vi "MARS_Global_var.vi"() -> ()   [LabVIEW 2015]
panel:
  in  "Fit Selection":bool
  in  "Int. Selector":bool caption="Integral Selector"
  in  "Select":bool
  in  "lower limit":i32
  in  "upper limit":i32
  in  "Listbox":i32[](array[numeric])
  out "Meas. Duration":dbl format="%^#.3g"
  out "2nd Integr.":dbl format="%^#.2g"
  out "1st Integr.":dbl format="%^#.2g"
  out "Trigger Level":dbl format="%#.3p"
  in  "Fit index":i32=1
  out "FoM":dbl
  out "Histogram":i32[][](graph)
  in  "Spectrum sel. 2":bool
  out "Discr. Spectrum":i32[][](array[numeric])
  out "Neutron Counts %":dbl format="%#.2f"
  out "Gamma Counts %":dbl format="%#.2f"
  out "Isotope Spectrum":i32[][](array[numeric])
  in  "Spectr. Sel.":bool
  out "Int Graph":i32[][](graph)
  out "Scatter":T1(graph) caption="Scatter Plot"
  out "Spectrum":i32[][](graph)
  out "Gamma Counts":i32
  out "Neutron Counts":i32
  out "Total Counts":i32
  in  "Fit Slope":dbl
  in  "Fit Offset":dbl
  out "Total Int. Auto":i32[][][](array[numeric])
  out "Tail Int. Auto":i32[][][](array[numeric])
  out "Total Integral":i32[](array[numeric])
  out "Tail Integral":i32[](array[numeric])
  out "Prog Ind":bool caption="CyUSB\nProg."
  out "Config Ind":bool caption="MB \nConfig."
  in  "Integ_per":cluster{dbl, dbl}(slide) caption="Duration of Integration (us)" scale=0.0..10.0
  in  "Error":errorcluster
  in  "Trig_thr":dbl(slide) caption="Trigger Threshold (V)" min=0.0 max=3.3 step=0.001 scale=0.0..3.3
  in  "CyUSB VISA":refnum<visa-resource-name>
  # "VISA Resource"
  # "Indicators"
  # "Configuration Data"
  # "Free Run Results Data"
  # "Auto Test Results Data"
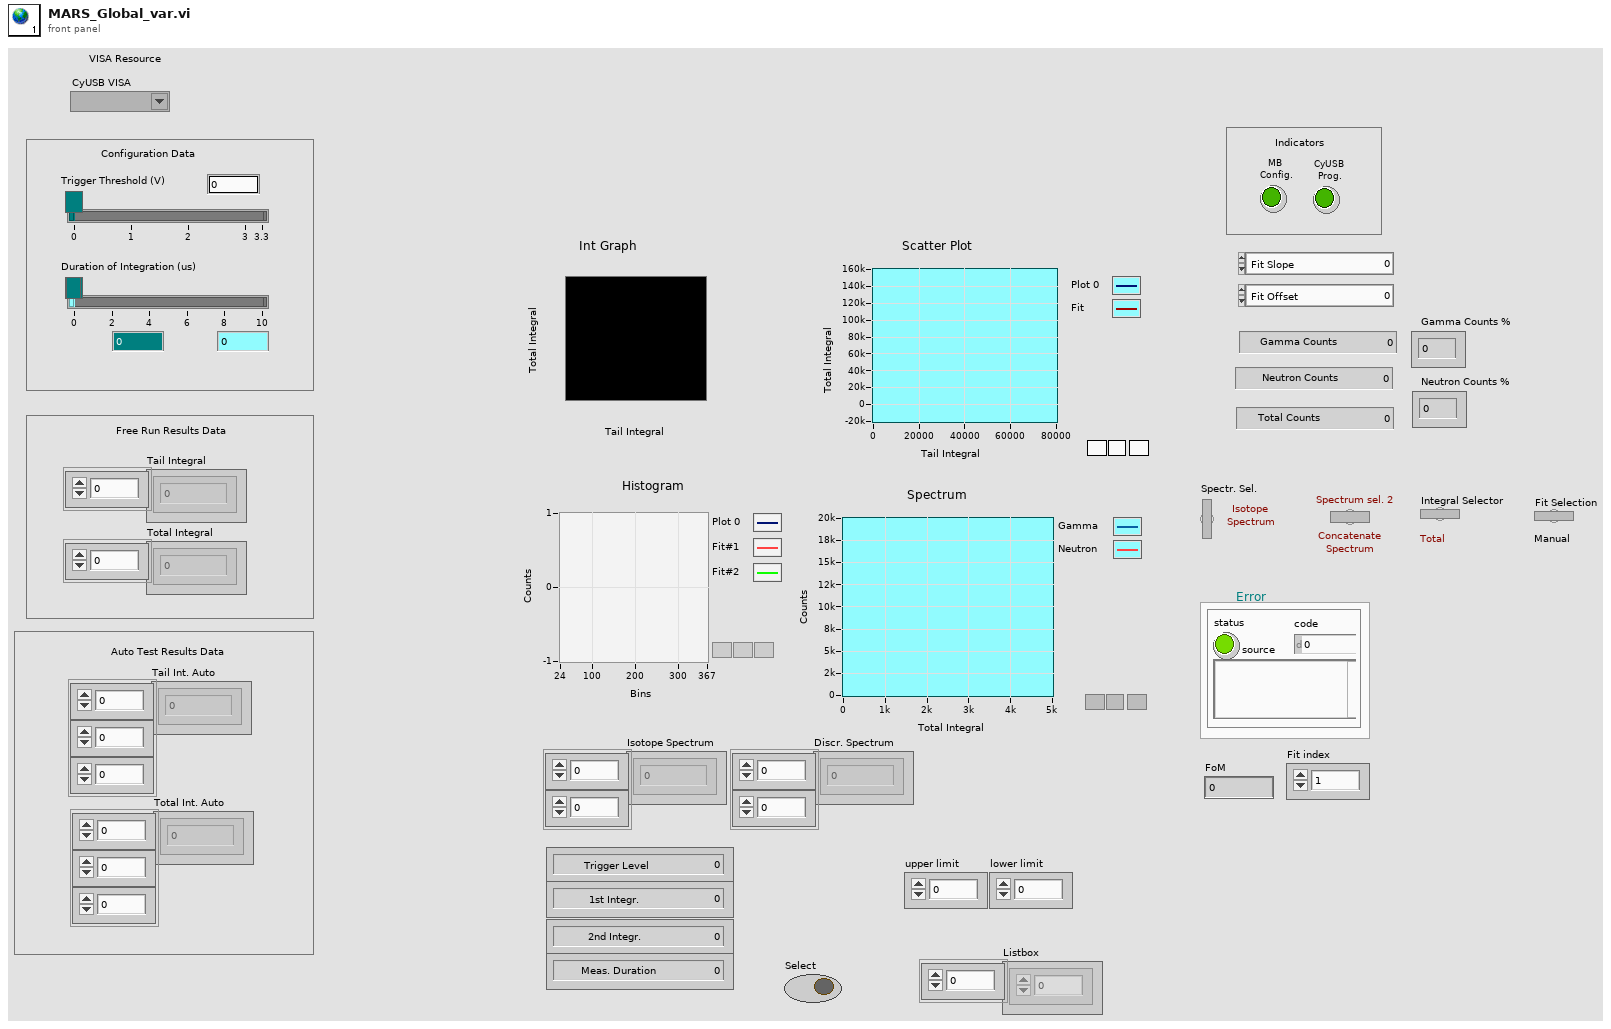
[diagram p1: front panel]
types:
  T1 = cluster{"Tail Integral":i32[], "Total Integral":dbl[]}[]
diagram:
